vi "shuttersOpen.vi"() -> ()   [LabVIEW 2017]
uses:
  globalDevices.vi
panel:
  out "*IDN?":string
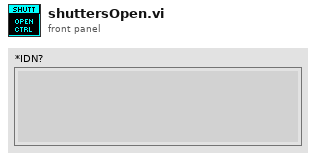
[diagram p1: front panel]
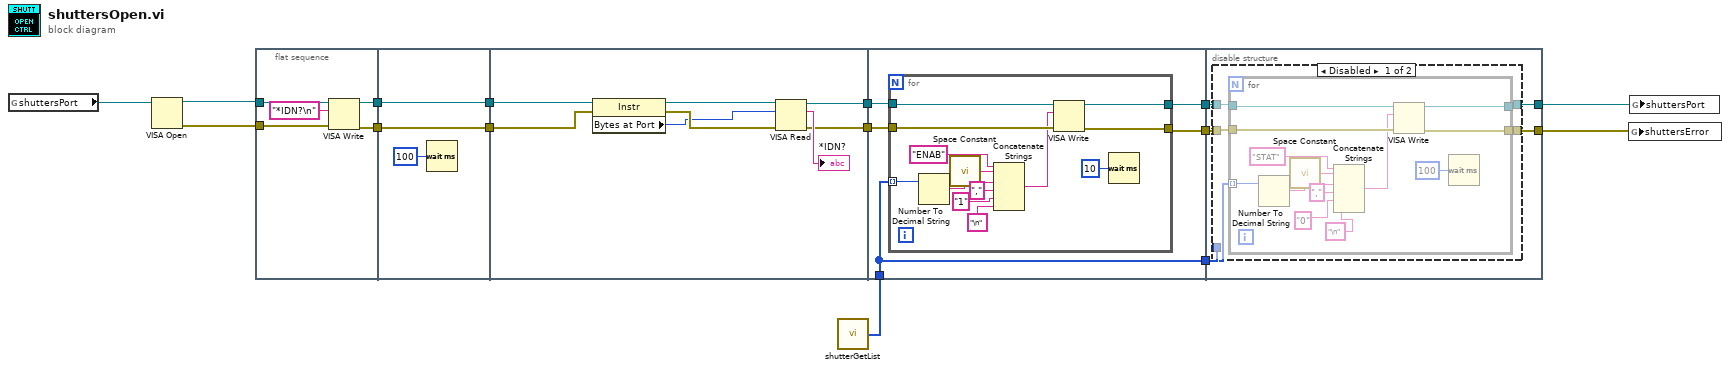
[diagram p0: block diagram]
diagram:
  n1 = global read "globalDevices.vi" "shuttersPort"() -> (w4:refnum<visa-resource-name>)
  n2 = VISA Open(VISA resource name=w4) -> (VISA resource name=w3:refnum<visa-resource-name>, error out=w2:errorcluster)  [unwired: 4 in]
  n3 = flat-sequence {
    tunnel: w3 -> [w20]
    tunnel: [w18] -> w14
    tunnel: [w17] -> w13
    tunnel: w2 -> [w16]
    tunnel: [w22] -> w15
    tunnel: w14 -> [w22]
    tunnel: w13 -> [w21]
    tunnel: [w21] -> w12
    tunnel: w15 -> [w27]
    tunnel: w12 -> [w28]
    tunnel: [w30] -> w11
    tunnel: [w29] -> w10
    tunnel: w11 -> [w36]
    tunnel: w10 -> [w35]
    tunnel: w1 -> [w32]
    tunnel: [w34] -> w9
    tunnel: [w33] -> w8
    tunnel: [w32] -> w7
    tunnel: w9 -> [w53]
    tunnel: w8 -> [w54]
    tunnel: w7 -> [w52]
    tunnel: [w51] -> w6
    tunnel: [w50] -> w5
    frame #0 {
      n4 = VISA Write(VISA resource name=w20, write buffer="*IDN?\n", error in (no error)=w16) -> (VISA resource name out=w18:refnum<visa-resource-name>, error out=w17:errorcluster)  [unwired: 1 out]
    }
    frame #1 {
      n5 = Wait (ms)(milliseconds to wait=u32 100) -> ()  [unwired: 1 out]
    }
    frame #2 {
      n6 = property class="Instr"(reference=w27, error in=w28) -> (reference out=w26:refnum<visa-resource-name>, error out=w25:errorcluster, "Bytes at Port"=w24:u32)
      n7 = VISA Read(VISA resource name=w26, byte count=w24, error in (no error)=w25) -> (VISA resource name out=w30:refnum<visa-resource-name>, read buffer=→"*IDN?":string, error out=w29:errorcluster)  [unwired: 1 out]
    }
    frame #3 {
      n8 = for {
        tunnel: w36 -> [w43]
        tunnel: w35 -> [w42]
        tunnel: w32 -> [w49] mode=indexing
        tunnel: [w39] -> w34
        tunnel: [w38] -> w33
        n9 = Number To Decimal String(number=w49) -> (decimal integer string=w46:string)  [unwired: 1 in]
        n10 = call <vilib>:"Space Constant.vi"() -> ("String"=w48:string)
        n11 = Concatenate Strings("ENAB", w48, w46, "," ("string"), "1" ("string"), "\n") -> (w41:string)
        n12 = VISA Write(VISA resource name=w43, write buffer=w41, error in (no error)=w42) -> (VISA resource name out=w38:refnum<visa-resource-name>, error out=w39:errorcluster)  [unwired: 1 out]
        n13 = Wait (ms)(milliseconds to wait=u32 10) -> ()  [unwired: 1 out]
      }
    }
    frame #4 {
      n14 = disable-structure shown="Disabled" {
        disable-tunnel: w54 -> [w59 _]
        disable-tunnel: w53 -> [w58 _]
        disable-tunnel: w52 -> [w57 _]
        disable-tunnel: [w56 _] -> w51
        disable-tunnel: [w55 _] -> w50
        frame Disabled {
          n15 = for {
            tunnel: w59 -> [w66]
            tunnel: w58 -> [w65]
            tunnel: w57 -> [w72] mode=indexing
            tunnel: [w62] -> w55
            tunnel: [w61] -> w56
            n16 = Number To Decimal String(number=w72) -> (decimal integer string=w69:string)  [unwired: 1 in]
            n17 = call <vilib>:"Space Constant.vi"() -> ("String"=w71:string)
            n18 = Concatenate Strings("STAT", w71, w69, "," ("string"), "0" ("string"), "\n") -> (w64:string)
            n19 = VISA Write(VISA resource name=w66, write buffer=w64, error in (no error)=w65) -> (VISA resource name out=w61:refnum<visa-resource-name>, error out=w62:errorcluster)  [unwired: 1 out]
            n20 = Wait (ms)(milliseconds to wait=u32 100) -> ()  [unwired: 1 out]
          }
        }
        frame Enabled {
        }
      }
    }
  }
  n21 = call "shutterGetList.vi"() -> ("list of shutters"=w1:i32[])  [unwired: 1 in]
  n22 = global write "globalDevices.vi" "shuttersError"(w5) -> ()
  n23 = global write "globalDevices.vi" "shuttersPort"(w6) -> ()
